vi "transform.vi"(6 "SpaceVector.lvclass":refnum<class "SpaceVector.lvclass">, 7 "zoom":dbl=1.0, 8 "error in (no error)":errorcluster, 9 "x angle (psi)":dbl[unit], 10 "z angle (phi)":dbl[unit], 11 "TrajectoryMG100122GenericFPGA in":refnum<class "TrajectoryMG100122GenericFPGA.lvclass">) -> (0 "error out":errorcluster, 3 "TrajectoryMG100122GenericFPGA out":refnum<class "TrajectoryMG100122GenericFPGA.lvclass">)   [LabVIEW 2010, in "TrajectoryMG100122GenericFPGA.lvclass"]
uses:
  TrajectoryMG100122GenericFPGA.lvclass
  common/classes/SpaceVector/SpaceVector/SpaceVector.lvclass
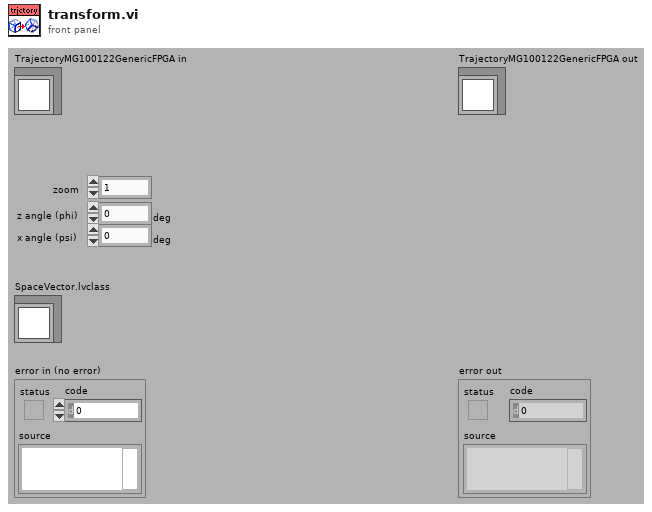
[diagram p1: front panel]
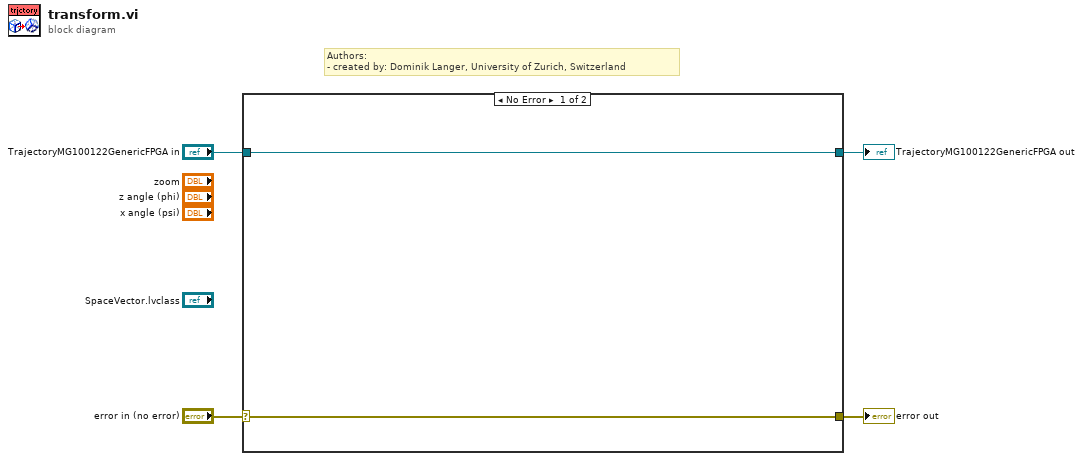
[diagram p0: block diagram]
diagram:
  # "Authors: \n- created by: Dominik Langer, University of Zurich, Switzerland"
  n1 = case shown="No Error" "error in (no error)" {
    selector: "error in (no error)" -> [w5 w8]
    tunnel: [w5 w8] -> w3
    tunnel: [w6 w7] -> w1
    tunnel: "TrajectoryMG100122GenericFPGA in" -> [w6 w7]
    frame No Error {
    }
    frame Error {
    }
  }
  "error out" <- w3
  "TrajectoryMG100122GenericFPGA out" <- w1
